vi "Command No-Op.vi"(7 "Startup":bool) -> (4 "Reint":bool, 6 "Completed":bool)   [LabVIEW 2017]
uses:
  Command Execution State.ctl
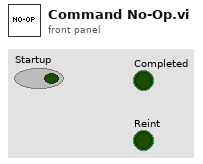
[diagram p1: front panel]
types:
  T1 = typedef "Command Execution State.ctl" = enum16{"Initialize", "Execute", "Finish"}
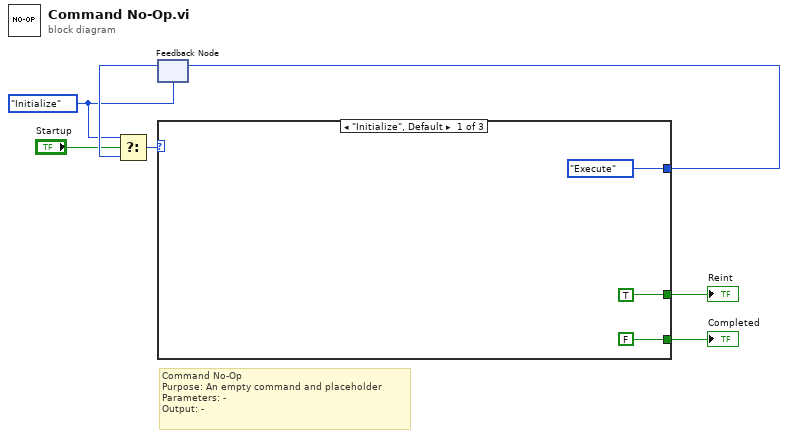
[diagram p0: block diagram]
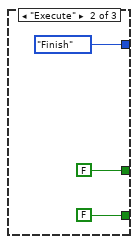
[diagram p2: hidden frame]
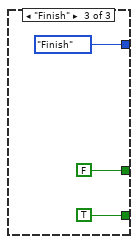
[diagram p3: hidden frame]
diagram:
  w4 = Command_Execution_State."Initialize" ("Play State")
  # "Command No-Op\nPurpose: An empty command and placeholder\nParameters: -\nOutput: -"
  n1 = feedback #1(w4) -> (w5:T1)
  n2 = Select(t=w4, s="Startup", f=w5) -> (s? t:f=w7:T1)
  n3 = case shown="\"Initialize\", Default" w7 {
    tunnel: [Command_Execution_State."Execute" ("Play State") Command_Execution_State."Finish" ("Play State") Command_Execution_State."Finish" ("Play State")] -> w6
    tunnel: [FALSE FALSE TRUE] -> w3
    tunnel: [TRUE FALSE FALSE] -> w1
    frame "Initialize", Default {
    }
    frame "Execute" {
    }
    frame "Finish" {
    }
  }
  "Completed" <- w3
  "Reint" <- w1
  n4 = feedback-in #1(w6) -> ()
